vi "多参数状态告警区读取.vi"(8 "Error in":errorcluster caption="Error in (no error)") -> (0 "error out":errorcluster, 2 "状态告警块":T1, 3 "添加的数组":string[][](array[string]))   [LabVIEW 2016, in "斯坦道仪器.lvlib"]
panel:
  in  "状态告警区":i32(listbox)
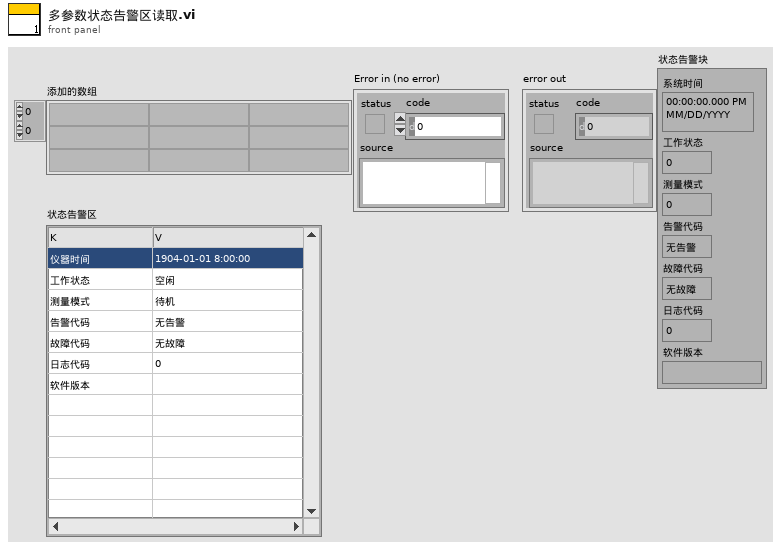
[diagram p1: front panel]
types:
  T1 = cluster{"系统时间":timestamp, "工作状态":u16, "测量模式":u16, "告警代码":enum16{"无告警", "缺试剂告警", "缺水样告警", "缺蒸馏水告警", "缺标液告警", "仪表漏液告警", "标定异常告警", "超量程告警", "加热异常", "低试剂预警", "超上限告警", "超下限告警", "仪表内部其他异常", "滴定异常告警", "电极异常告警", "量程切换告警", "参数设置告警", "PH电极电位异常", "电导率电极异常", "浊度光度异常", "溶解氧电极异常", "溶解氧光强异常", "温度异常告警", "PH异常告警", "溶解氧异常告警", "电导率异常告警", "浊度异常告警", "叶绿素异常告警", "藻密度异常告警", "蓝绿藻异常告警", "ORP异常告警", "氨氮异常告警", "清洁刷异常告警", "SD卡异常告警", "蓝牙异常告警", "Wifi异常告警", "流程异常告警"}, "故障代码":enum16{"无故障", "电机故障", "温度故障", "通讯故障", "滴定故障"}, "日志代码":u16, "软件版本":string}
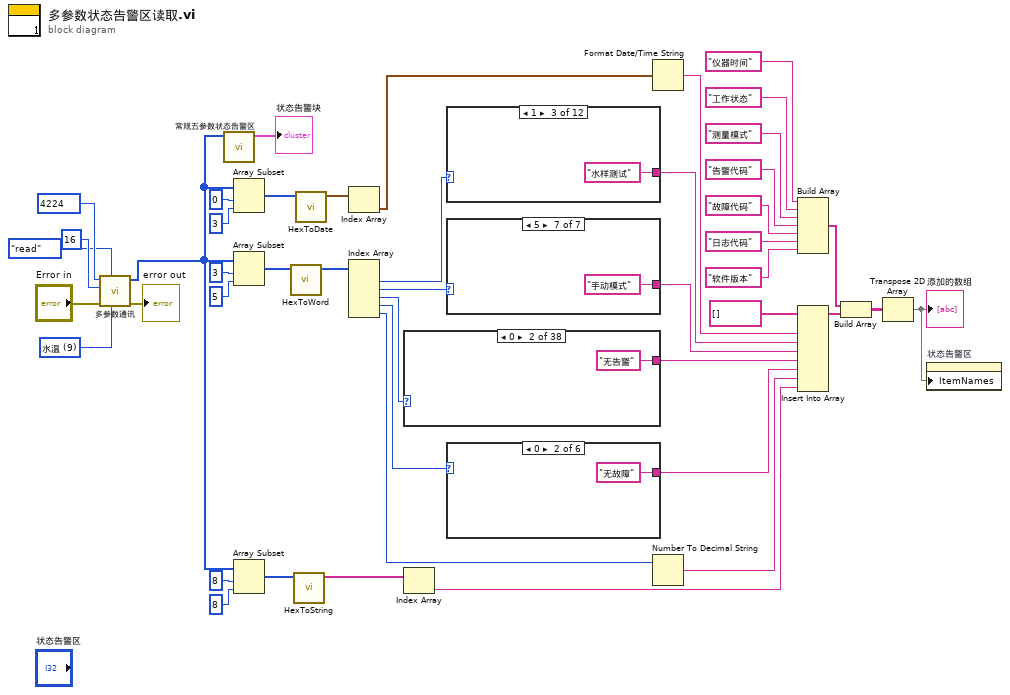
[diagram p0: block diagram]
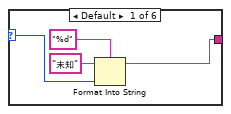
[diagram p2: hidden frame]
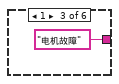
[diagram p3: hidden frame]
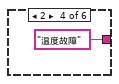
[diagram p4: hidden frame]
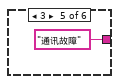
[diagram p5: hidden frame]
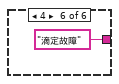
[diagram p6: hidden frame]
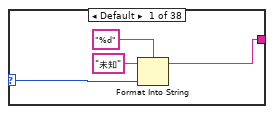
[diagram p7: hidden frame]
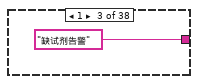
[diagram p8: hidden frame]
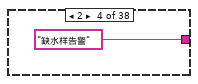
[diagram p9: hidden frame]
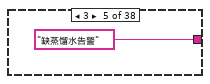
[diagram p10: hidden frame]
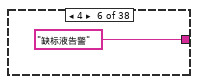
[diagram p11: hidden frame]
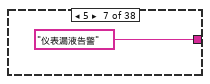
[diagram p12: hidden frame]
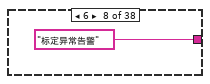
[diagram p13: hidden frame]
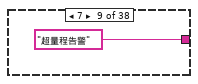
[diagram p14: hidden frame]
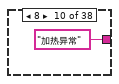
[diagram p15: hidden frame]
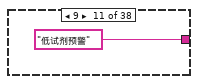
[diagram p16: hidden frame]
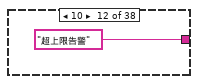
[diagram p17: hidden frame]
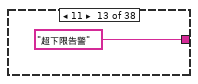
[diagram p18: hidden frame]
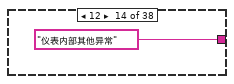
[diagram p19: hidden frame]
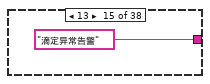
[diagram p20: hidden frame]
diagram:
  w2 = u16 9 items=["氨氮"=3, "水温"=9, "pH值"=10, "溶解氧"=11, "电导率"=12, "浊度"=13, "叶绿素a"=14, "藻密度"=15, "蓝绿藻"=16, "氧化还原电位"=17, "溶解氧%"=18, "盐度"=19] ("探头选择")
  n1 = call "多参数通讯.vi"("Slave ID"=w2, "STEP"=enum16{"open", "read", "write", "close"}."read", "Error in"="Error in", "quantity"=u16 16, "starting address"=u16 4224) -> ("error out"=→"error out":errorcluster, "Registers"=w4:u16[])  [unwired: 4 in, 1 out]
  n2 = call "常规五参数状态告警区.vi"("数组"=w4) -> ("状态告警区"=→"状态告警块":T1)  [unwired: 10 in]
  n3 = Array Subset(array=w4, index=0 ("索引"), length=3 ("长度")) -> (w29:u16[])
  n4 = Array Subset(array=w4, index=3 ("索引"), length=5 ("长度")) -> (w25:u16[])
  n5 = Array Subset(array=w4, index=8 ("索引"), length=8 ("长度")) -> (w23:u16[])
  n6 = call "HexToWord.vi"("数组"=w25) -> ("WORD"=w16:u16[])  [unwired: 10 in]
  n7 = call "HexToString.vi"("数组"=w23) -> ("STRING"=w21:string[])  [unwired: 10 in]
  n8 = call "HexToDate.vi"("数组"=w29) -> ("DATE"=w26:timestamp[])  [unwired: 10 in]
  n9 = Index Array(array=w26) -> (element=w20:timestamp)  [unwired: 1 in]
  n10 = Index Array(array=w16) -> (element #1=w15:u16, element #2=w14:u16, element #3=w12:u16, element #4=w13:u16, element #5=w11:u16)  [unwired: 5 in]
  n11 = case shown="0" w12 {
    selector: w12 -> [w47 _ _ _ _ _ _ _ _ _ _ _ _ _ _ _ _ _ _ _ _ _ _ _ _ _ _ _ _ _ _ _ _ _ _ _ _ _]
    tunnel: [w46 "无告警" "缺试剂告警" "缺水样告警" "缺蒸馏水告警" "缺标液告警" "仪表漏液告警" "标定异常告警" "超量程告警" "加热异常" "低试剂预警" "超上限告警" "超下限告警" "仪表内部其他异常" "滴定异常告警" "电极异常告警" "量程切换告警" "参数设置告警" "PH电极电位异常" "电导率电极异常" "浊度光度异常" "溶解氧电极异常" "溶解氧光强异常" "温度异常告警" "PH异常告警" "溶解氧异常告警" "电导率异常告警" "浊度异常告警" "叶绿素异常告警" "藻密度异常告警" "蓝绿藻异常告警" "ORP异常告警" "氨氮异常告警" "清洁刷异常告警" "SD卡异常告警" "蓝牙异常告警" "WiFi异常告警" "流程异常告警"] -> w7
    frame Default {
      n12 = Format Into String(format string="%d" ("格式字符串"), initial string="未知" ("工作状态"), w47) -> (resulting string=w46:string)  [unwired: 1 in, 1 out]
    }
    frame 0 {
    }
    frame 1 {
    }
    frame 2 {
    }
    frame 3 {
    }
    frame 4 {
    }
    frame 5 {
    }
    frame 6 {
    }
    frame 7 {
    }
    frame 8 {
    }
    frame 9 {
    }
    frame 10 {
    }
    frame 11 {
    }
    frame 12 {
    }
    frame 13 {
    }
    frame 14 {
    }
    frame 15 {
    }
    frame 16 {
    }
    frame 17 {
    }
    frame 18 {
    }
    frame 19 {
    }
    frame 20 {
    }
    frame 21 {
    }
    frame 22 {
    }
    frame 23 {
    }
    frame 24 {
    }
    frame 25 {
    }
    frame 26 {
    }
    frame 27 {
    }
    frame 28 {
    }
    frame 29 {
    }
    frame 30 {
    }
    frame 31 {
    }
    frame 32 {
    }
    frame 33 {
    }
    frame 34 {
    }
    frame 35 {
    }
    frame 36 {
    }
  }
  n13 = Index Array(array=w21) -> (element=w10:string)  [unwired: 1 in]
  n14 = case shown="1" w15 {
    selector: w15 -> [w87 _ _ _ _ _ _ _ _ _ _ _]
    tunnel: [w88 "空闲" ("工作状态") "水样测试" ("工作状态") "标样核查" ("工作状态") "零点核查" ("工作状态") "跨度核查" ("工作状态") "空白测试" ("工作状态") "平行样测试" ("工作状态") "加标回收" ("工作状态") "空白校准" ("工作状态") "标样校准" ("工作状态") "初始化" ("工作状态")] -> w6
    frame Default {
      n15 = Format Into String(format string="%d" ("格式字符串"), initial string="未知" ("工作状态"), w87) -> (resulting string=w88:string)  [unwired: 1 in, 1 out]
    }
    frame 0 {
    }
    frame 1 {
    }
    frame 2 {
    }
    frame 3 {
    }
    frame 4 {
    }
    frame 5 {
    }
    frame 6 {
    }
    frame 7 {
    }
    frame 8 {
    }
    frame 9 {
    }
    frame 10 {
    }
  }
  n16 = case shown="5" w14 {
    selector: w14 -> [w102 _ _ _ _ _ _]
    tunnel: [w103 "待机" "连续模式" "周期模式" "定点模式" "受控模式" "手动模式"] -> w5
    frame Default {
      n17 = Format Into String(format string="%d" ("格式字符串"), initial string="未知" ("工作状态"), w102) -> (resulting string=w103:string)  [unwired: 1 in, 1 out]
    }
    frame 0 {
    }
    frame 1 {
    }
    frame 2 {
    }
    frame 3 {
    }
    frame 4 {
    }
    frame 5 {
    }
  }
  n18 = case shown="0" w13 {
    selector: w13 -> [w113 _ _ _ _ _]
    tunnel: [w112 "无故障" "电机故障" "温度故障" "通讯故障" "滴定故障"] -> w8
    frame Default {
      n19 = Format Into String(format string="%d" ("格式字符串"), initial string="未知" ("工作状态"), w113) -> (resulting string=w112:string)  [unwired: 1 in, 1 out]
    }
    frame 0 {
    }
    frame 1 {
    }
    frame 2 {
    }
    frame 3 {
    }
    frame 4 {
    }
  }
  n20 = Format Date/Time String(seconds (now)=w20) -> (date/time string=w18:string)  [unwired: 2 in]
  n21 = Number To Decimal String(number=w11) -> (decimal integer string=w9:string)  [unwired: 1 in]
  n22 = Build Array("仪器时间", "工作状态", "测量模式", "告警代码", "故障代码", "日志代码", "软件版本") -> (w36:string[])
  n23 = Insert Into Array(array=string[] [] ("数组"), new element #1=w18, new element #2=w6, new element #3=w5, new element #4=w7, new element #5=w8, new element #6=w9, new element #7=w10) -> (w17:string[])  [unwired: 1 in]
  n24 = Build Array(w36, w17) -> (w35:string[][])
  n25 = Transpose 2D Array(2D array=w35) -> (transposed array=w34:string[][])
  "添加的数组" <- w34
  n26 = property on="状态告警区" class="MCListbox (严格)"("ItemNames"=w34) -> ()  [unwired: 2 in, 2 out]
